vi "Ancestor Classes.vi"(8 "error in (no error)":errorcluster, 11 "Section 2 in":refnum<class "Section 2.lvclass">) -> (0 "error out":errorcluster, 1 "Ancestor Classes":string[](array[string]), 2 "Ancestor Class Pathes":path[](array[path]), 3 "Section 2 out":refnum<class "Section 2.lvclass">)   [LabVIEW 2012, in "LVOOP Introduction.lvlib" / "Section 2.lvclass"]
doc: "This VI returns array of all ancestor classes and their pathes."
uses:
  Section 2.lvclass
  Configuration/Classes/Section/Section.lvclass
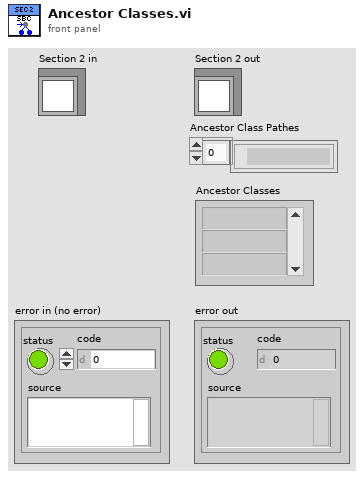
[diagram p1: front panel]
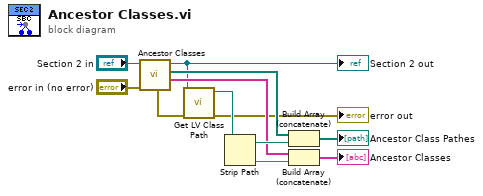
[diagram p0: block diagram]
diagram:
  n1 = call-parent "Ancestor Classes.vi"("error in (no error)"="error in (no error)", "Section in"="Section 2 in") -> ("error out"=w10:errorcluster, "Ancestor Classes"=w7:string[], "Ancestor Class Pathes"=w8:path[], "Section out"=w3:refnum<class "Section 2.lvclass">)  [unwired: 6 in]
  "Section 2 out" <- w3
  n2 = call <vilib>:"Get LV Class Path.vi"("error in (no error)"=w10, "object"=w3) -> ("error out"=→"error out":errorcluster, "class path"=w9:path)  [unwired: 8 in]
  n3 = Strip Path(path=w9) -> (stripped path=w11:path, name=w12:string)
  n4 = Build Array (concatenate)(w8, w11) -> (→"Ancestor Class Pathes":path[])
  n5 = Build Array (concatenate)(w7, w12) -> (→"Ancestor Classes":string[])
